vi "Collect&Filter.vi"(9 "chart":dbl[](array[numeric]), 10 "Boolean":bool, 11 "Numeric in":i32) -> (1 "Collected Signals":dynamicdata(waveform), 2 "Numeric out":i32, 3 "Array Size":u32, 4 "Filtered X":dbl[](array[numeric]))   [LabVIEW 2021]
uses:
  <vilib>/Analysis/3filter.llb/Butterworth Filter (DBL).vi
  <vilib>/Analysis/NI_AALBase.lvlib
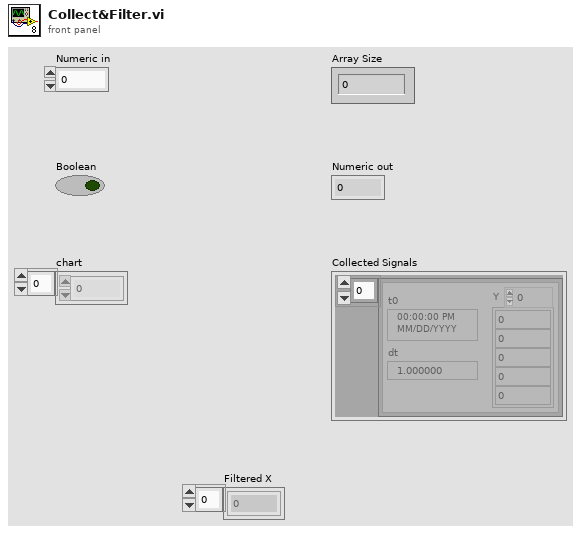
[diagram p1: front panel]
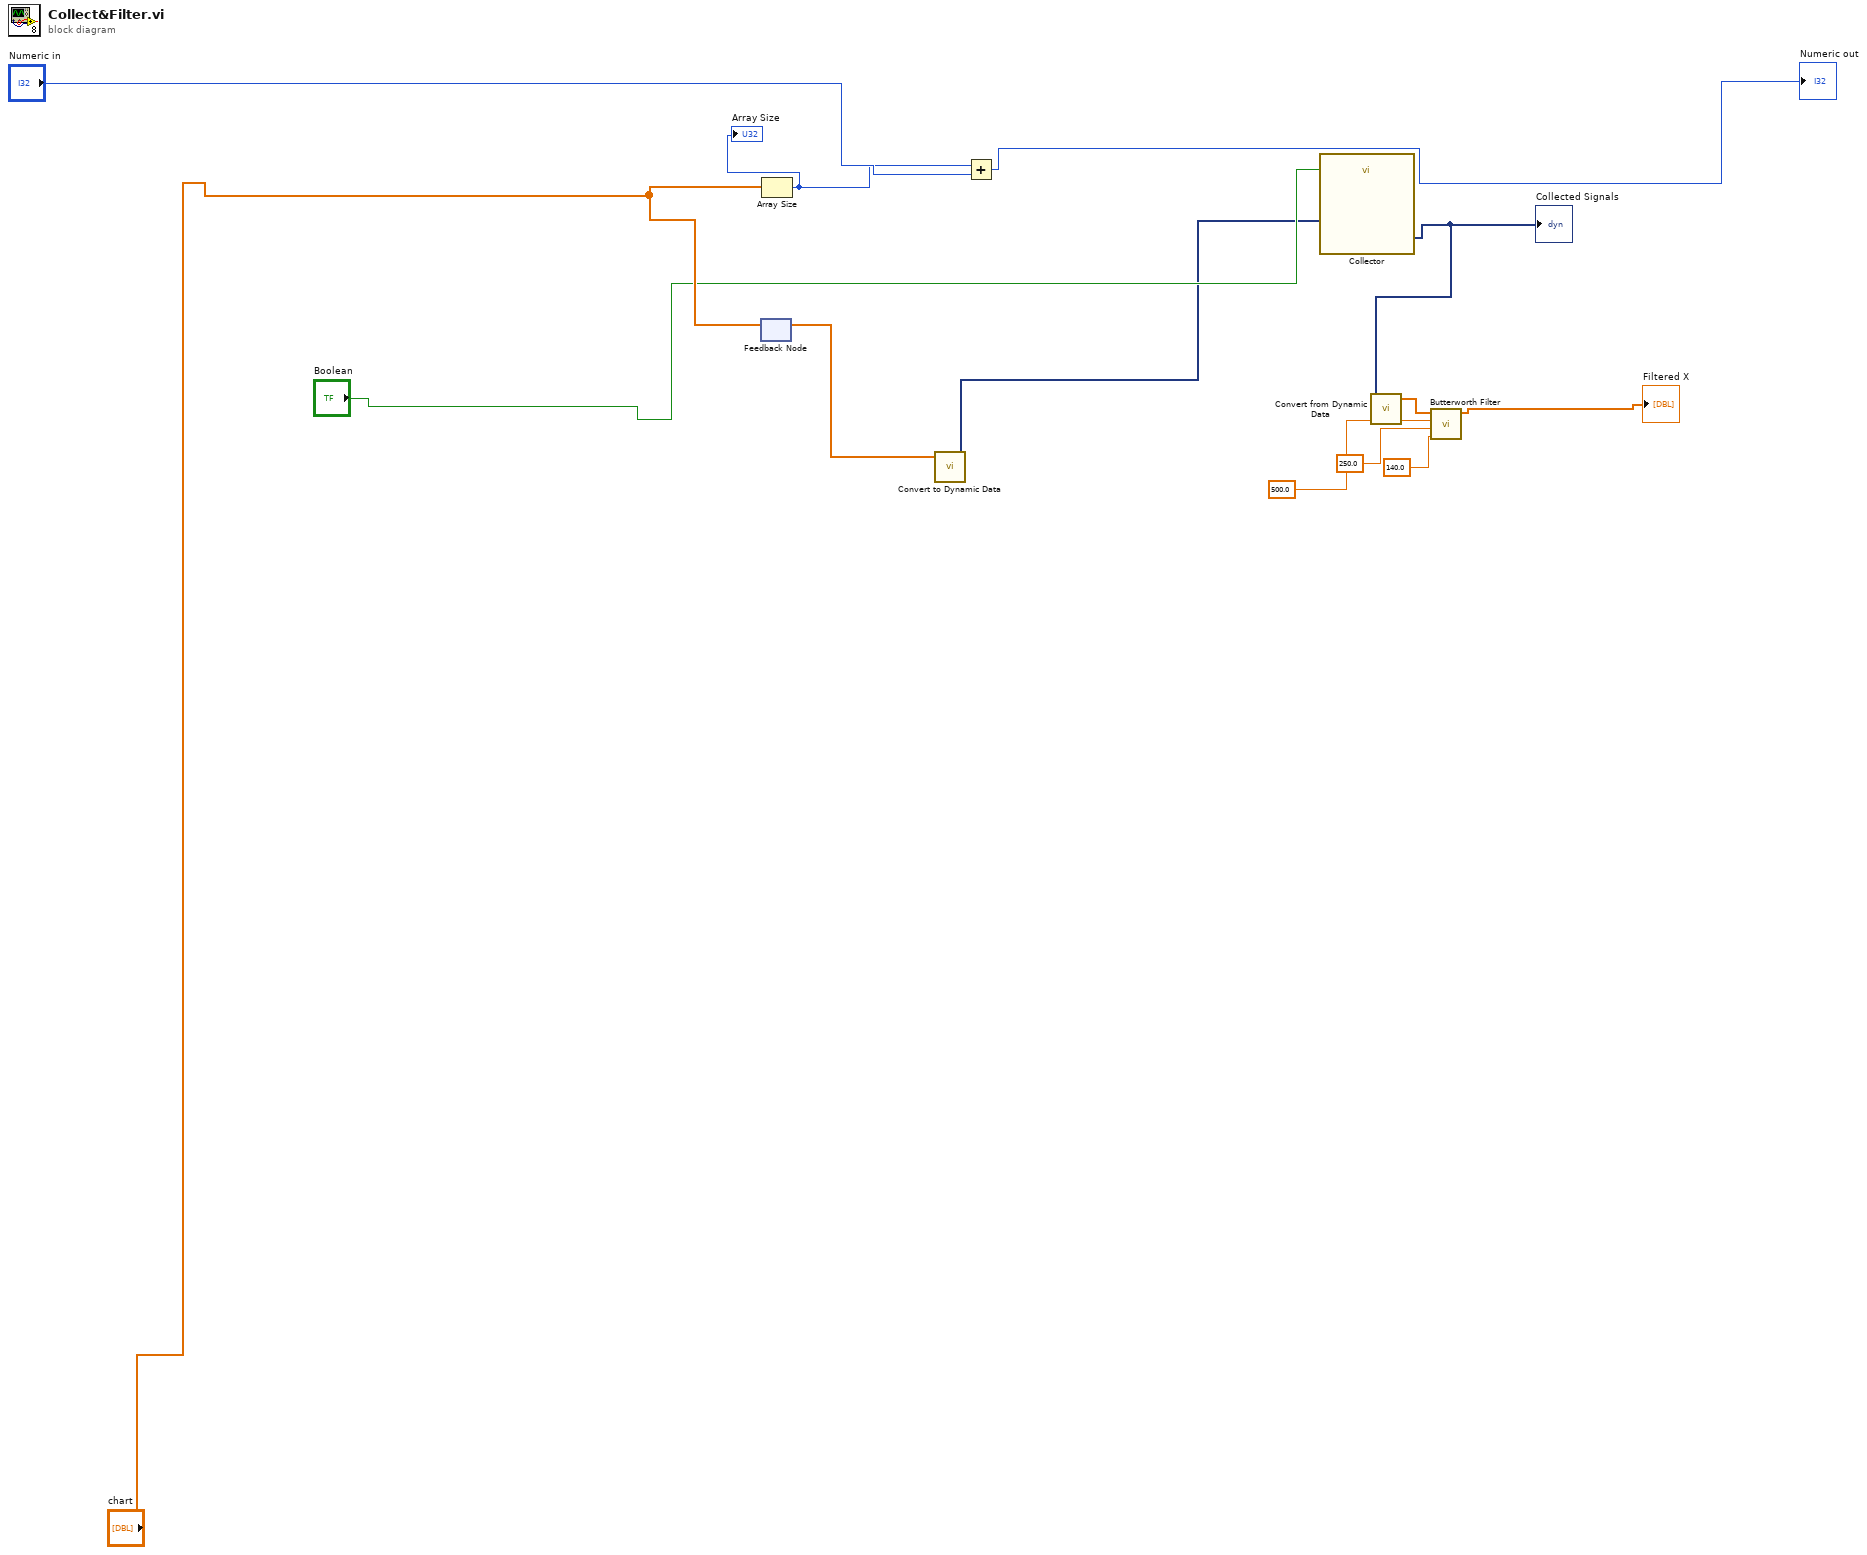
[diagram p0: block diagram]
diagram:
  n1 = feedback #1() -> (w7:dbl[])  [unwired: 1 in]
  n2 = feedback-in #1("chart") -> ()
  n3 = Array Size(array="chart") -> (size(s)=w8:i32)
  "Array Size" <- w8
  n4 = call "Convert to Dynamic Data"("Array"=w7) -> ("Dynamic Data Type"=w6:dynamicdata)  [unwired: 3 in]
  n5 = Add(x=w8, y="Numeric in") -> (x+y=→"Numeric out":i32)
  n6 = call "Collector"("Enable"="Boolean", "Signals"=w6) -> ("Collected Signals"=w5:dynamicdata)  [unwired: 8 in, 1 out]
  "Collected Signals" <- w5
  n7 = call "Convert from Dynamic Data"("Dynamic Data Type"=w5) -> ("Array"=w4:dbl[])  [unwired: 3 in]
  n8 = call-poly <vilib>:"Butterworth Filter.vi"("low cutoff freq: fl"=140.0, "high cutoff freq: fh"=250.0, "sampling freq: fs"=500.0, "X"=w4) -> ("Filtered X"=→"Filtered X":dbl[])  [unwired: 4 in, 1 out]
